vi "Save_Data.vi"(1 "Index":u16, 2 "Plot Type":T1=enum."Voltage trace") -> ()   [LabVIEW 2016]
uses:
  Controls/Graph_Type.ctl
  Controls/XY_Plot_Cluster.ctl
  Controls/Inst_type.ctl
  Globals/Meas_global.vi
  Globals/Plug_in_data_global.vi
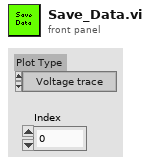
[diagram p1: front panel]
types:
  T1 = typedef "Graph_Type.ctl" = enum16{"Show no graph", "Voltage trace", "Velocity trace", "Vel histogram", "Spectrum", "f.E(f) v Log f", "Auto-Corr"}
  T2 = typedef "Analysis_info_cluster.ctl" = cluster{"Colour":u32, "Inst type":T3, "Inst name":string, "Symbol":string, "Code name":string, "Extra Info":string, "Inst Array":T4, "Extra Titles":string[], "Extra Values":string[], "U":dbl, "u^2":dbl, "u^3":dbl, "u^4":dbl, "Skew_u":dbl, "Kurt_u":dbl, "Sd Error in Mean":dbl, "% u'/U":dbl, "X":dbl, "Y":dbl, "Z":dbl, "Timescale integral Estimate":dbl, "Sd Error in Variance":dbl, "Calib File":path, "Calib Constants":dbl[], "Output Position":bool, "Full Stats":bool, "Av Sampling Rate":dbl, "Av No of Samples":dbl, "Total Meas Time (s)":dbl, "ADAM Ch Name":string, "Max value":dbl, "Min value":dbl}
  T3 = typedef "Inst_type.ctl" = enum16{"Propeller anemometer", "Raw voltage", "Pressure Transducer", "Pitot-static tube", "Preston tube", "Hot wire", "Cross wire 1", "Cross wire 2", "Generic Linear", "Generic Polynomial", "Generic BackPoly", "Fast FID", "Thermocouple", "Cold wire", "Pulsed Wire", "LDA Vel", "LDA Tran time", "LDA Arr time", "Microphone"}
  T4 = typedef "Instrument_Array.ctl" = enum16{"PWA", "LDA", "Analogue"}
  T5 = typedef "Post_Process.ctl" = enum16{"Take New Data", "Post Process Raw Data File"}
  T6 = typedef "XY_Plot_Cluster.ctl" = cluster{"First Name":string, "Second Name":string, "X axis name":string, "Y axis name":string, "X array":dbl[], "Y array":dbl[], "Weighting":dbl[]}
  T7 = typedef "Time_Trace_Cluster.ctl" = cluster{"Weighting":dbl[], "Time (s)":dbl[], "Voltage":dbl[], "Eng Values":dbl[]}
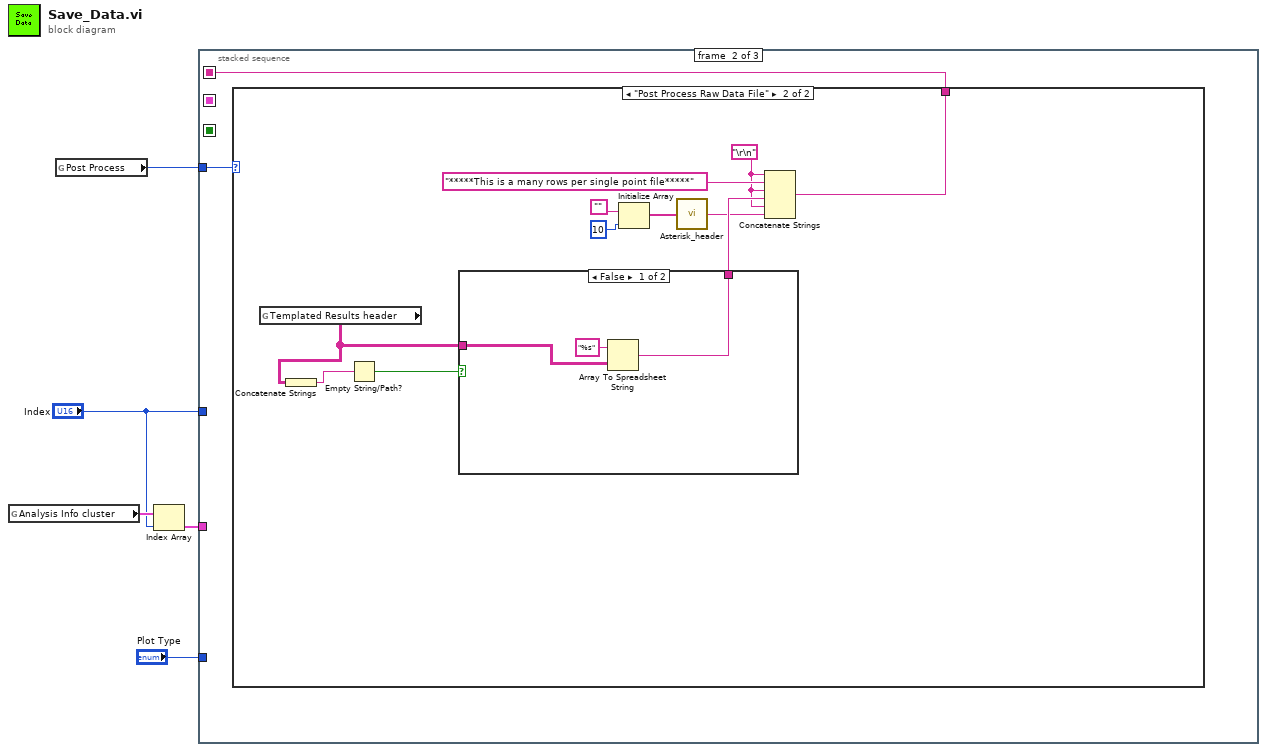
[diagram p0: block diagram]
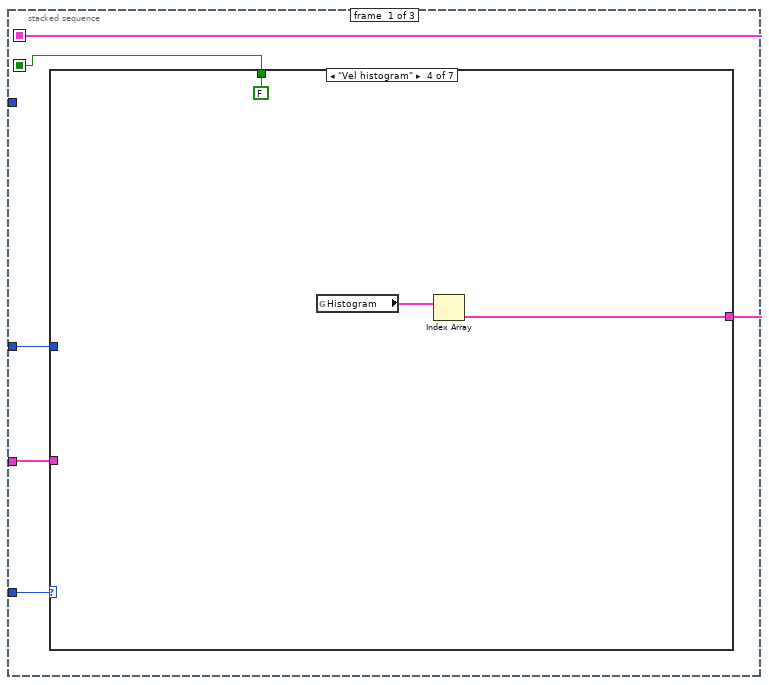
[diagram p2: hidden frame]
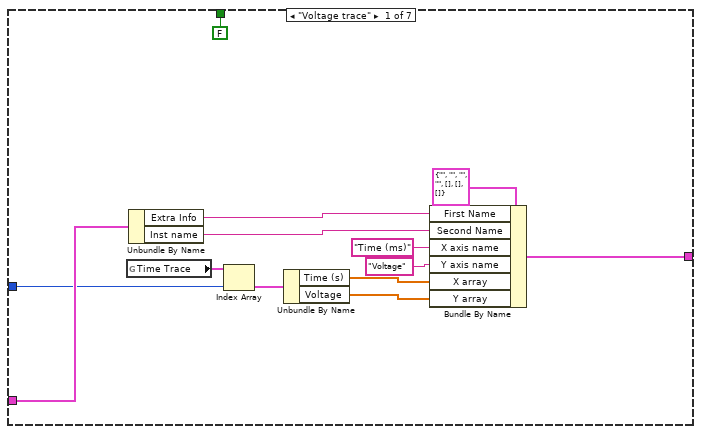
[diagram p3: hidden frame]
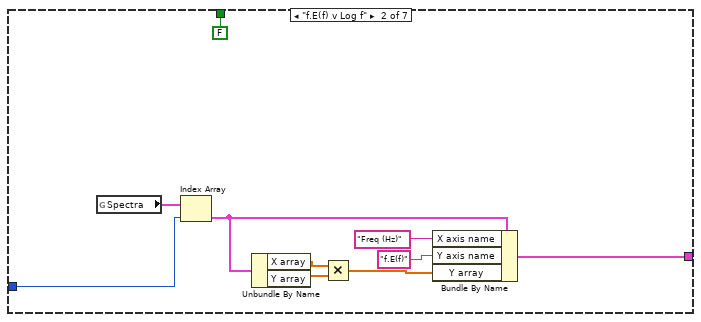
[diagram p4: hidden frame]
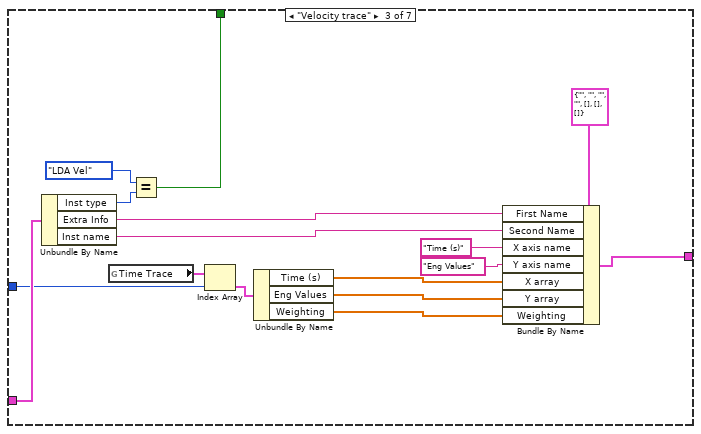
[diagram p5: hidden frame]
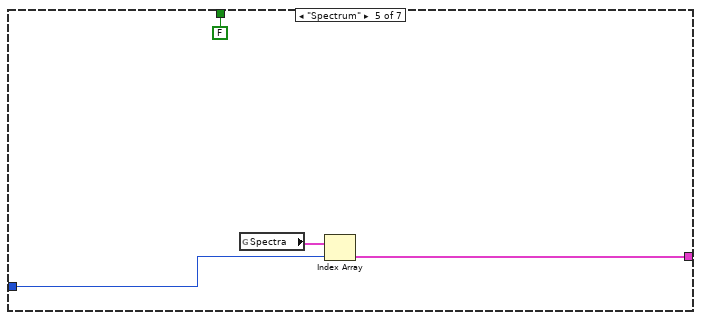
[diagram p6: hidden frame]
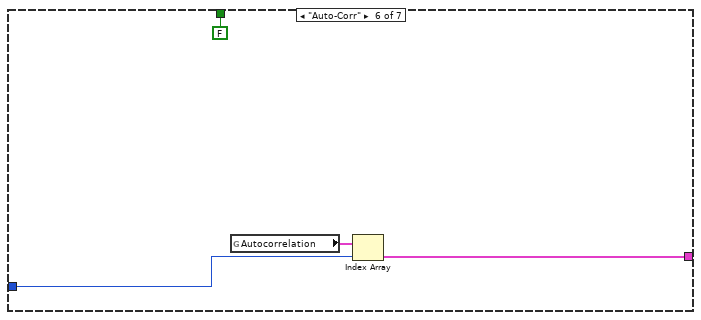
[diagram p7: hidden frame]
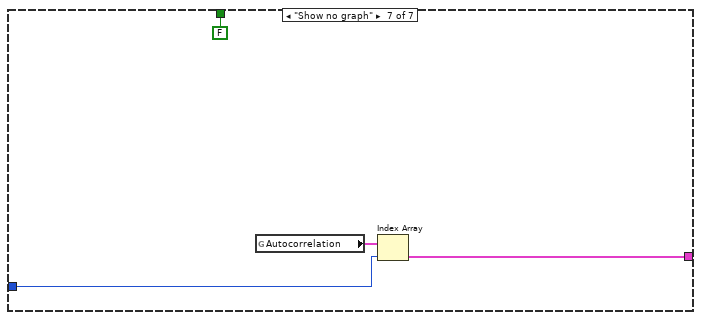
[diagram p8: hidden frame]
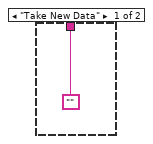
[diagram p9: hidden frame]
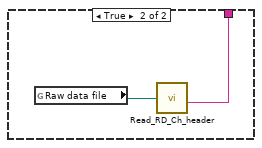
[diagram p10: hidden frame]
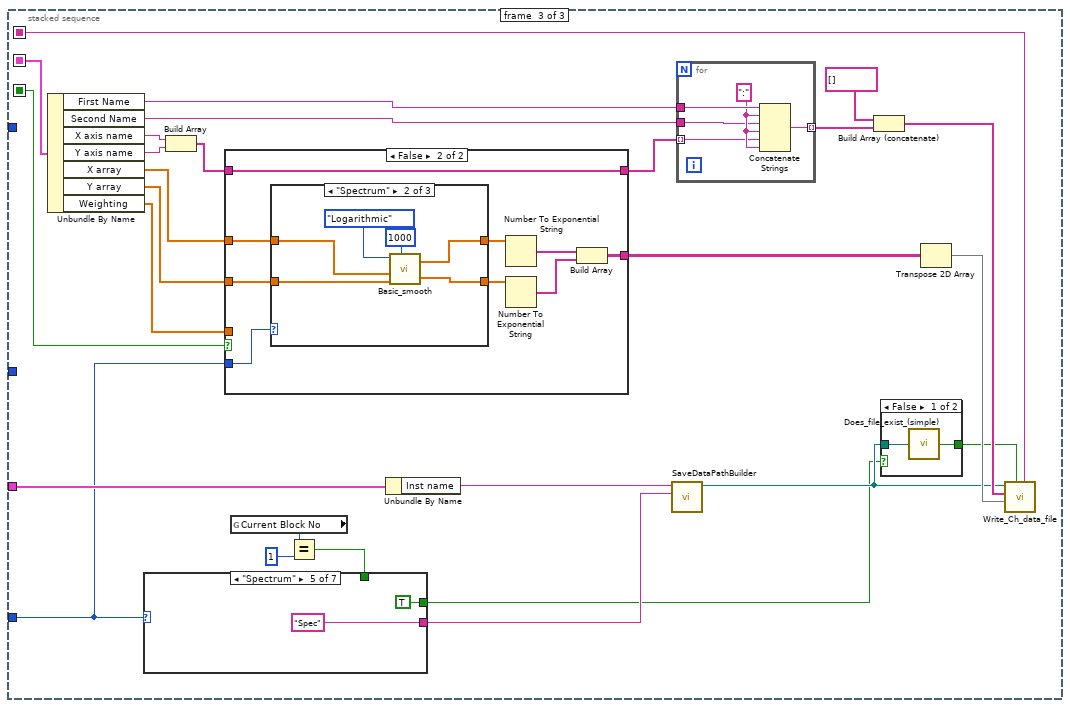
[diagram p11: hidden frame]
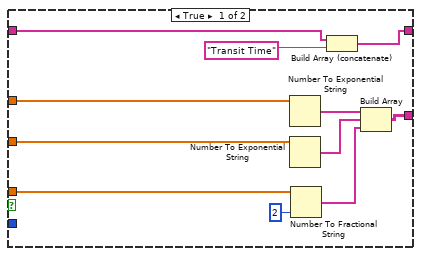
[diagram p12: hidden frame]
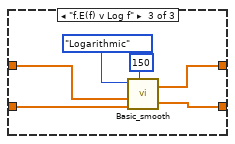
[diagram p14: hidden frame]
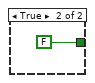
[diagram p15: hidden frame]
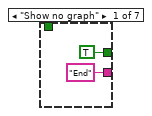
[diagram p16: hidden frame]
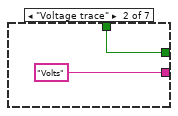
[diagram p17: hidden frame]
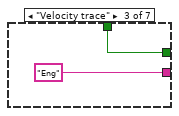
[diagram p18: hidden frame]
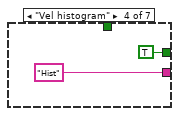
[diagram p19: hidden frame]
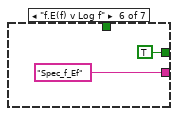
[diagram p20: hidden frame]
diagram:
  n1 = global read "Meas_global.vi" "Analysis Info cluster"() -> (w3:T2[])
  n2 = global read "Meas_global.vi" "Post Process"() -> (w4:T5)
  n3 = Index Array(array=w3, index="Index") -> (element=w2:T2)
  n4 = stacked-sequence {
    seq-local: [w8 _ _] -> [_ _ w95]
    seq-local: [_ w65 _] -> [_ _ w96]
    seq-local: [w6 _ _] -> [_ _ w91]
    tunnel: "Plot Type" -> [w10 _ w94]
    tunnel: w2 -> [w9 _ w104]
    tunnel: w4 -> [_ w66 _]
    tunnel: "Index" -> [w7 _ _]
    frame #0 {
      n5 = case shown="\"Vel histogram\"" w10 {
        tunnel: w9 -> [w23 _ w49 _ _ _ _]
        tunnel: [w18 w31 w44 w51 w56 w58 w62] -> w8
        tunnel: w7 -> [w16 w26 w41 _ w55 w59 w63]
        tunnel: [FALSE FALSE w34 FALSE FALSE FALSE FALSE] -> w6
        frame "Voltage trace" {
          n6 = global read "Meas_global.vi" "Time Trace"() -> (w17:T7[])
          n7 = Unbundle By Name(w23) -> ("Extra Info"=w22:string, "Inst name"=w21:string)
          n8 = Index Array(array=w17, index=w16) -> (element=w15:T7)
          n9 = Unbundle By Name(w15) -> ("Time (s)"=w14:dbl[], "Voltage"=w13:dbl[])
          n10 = Bundle By Name(cluster=T6 {"First Name"="", "Second Name"="", "X axis name"="", "Y axis name"="", "X array"=[], "Y array"=[], "Weighting"=[]} ("Spectra"), "First Name"=w22, "Second Name"=w21, "X axis name"="Time (ms)", "Y axis name"="Voltage", "X array"=w14, "Y array"=w13) -> (w18:T6)
        }
        frame "f.E(f) v Log f" {
          n11 = global read "Meas_global.vi" "Spectra"() -> (w27:T6[])
          n12 = Index Array(array=w27, index=w26) -> (element=w25:T6)
          n13 = Unbundle By Name(w25) -> ("X array"=w29:dbl[], "Y array"=w30:dbl[])
          n14 = Multiply(x=w29, y=w30) -> (x*y=w28:dbl[])
          n15 = Bundle By Name(cluster=w25, "X axis name"="Freq (Hz)", "Y axis name"="f.E(f)", "Y array"=w28) -> (w31:T6)
        }
        frame "Velocity trace" {
          n16 = Unbundle By Name(w49) -> ("Inst type"=w36:T3, "Extra Info"=w48:string, "Inst name"=w47:string)
          n17 = global read "Meas_global.vi" "Time Trace"() -> (w42:T7[])
          n18 = Equal?(x=Inst_type."LDA Vel" ("Inst type"), y=w36) -> (x = y?=w34:bool)
          n19 = Index Array(array=w42, index=w41) -> (element=w40:T7)
          n20 = Unbundle By Name(w40) -> ("Time (s)"=w39:dbl[], "Eng Values"=w38:dbl[], "Weighting"=w37:dbl[])
          n21 = Bundle By Name(cluster=T6 {"First Name"="", "Second Name"="", "X axis name"="", "Y axis name"="", "X array"=[], "Y array"=[], "Weighting"=[]} ("Spectra"), "First Name"=w48, "Second Name"=w47, "X axis name"="Time (s)", "Y axis name"="Eng Values", "X array"=w39, "Y array"=w38, "Weighting"=w37) -> (w44:T6)
        }
        frame "Vel histogram" {
          n22 = global read "Meas_global.vi" "Histogram"() -> (w52:T6[])
          n23 = Index Array(array=w52) -> (element=w51:T6)  [unwired: 1 in]
        }
        frame "Spectrum" {
          n24 = global read "Meas_global.vi" "Spectra"() -> (w54:T6[])
          n25 = Index Array(array=w54, index=w55) -> (element=w56:T6)
        }
        frame "Auto-Corr" {
          n26 = global read "Meas_global.vi" "Autocorrelation"() -> (w60:T6[])
          n27 = Index Array(array=w60, index=w59) -> (element=w58:T6)
        }
        frame "Show no graph" {
          n28 = global read "Meas_global.vi" "Autocorrelation"() -> (w64:T6[])
          n29 = Index Array(array=w64, index=w63) -> (element=w62:T6)
        }
      }
    }
    frame #1 {
      n30 = case shown="\"Post Process Raw Data File\"" w66 {
        tunnel: ["" w70] -> w65
        frame "Take New Data" {
        }
        frame "Post Process Raw Data File" {
          w71 = "\r\n"
          n31 = global read "Plug_in_data_global.vi" "Templated Results header"() -> (w69:string[][])
          n32 = Concatenate Strings(w69) -> (w68:string)
          n33 = Empty String/Path?(string/path=w68) -> (empty?=w77:bool)
          n34 = case shown="False" w77 {
            tunnel: [w79 w82] -> w76
            tunnel: w69 -> [w80 _]
            frame False {
              n35 = Array To Spreadsheet String(array=w80, 3:"%s" ("format string")) -> (spreadsheet string=w79:string)  [unwired: 1 out]
            }
            frame True {
              n36 = global read "Meas_global.vi" "Raw data file"() -> (w83:path)
              n37 = call "Read_RD_Ch_header.vi"("Raw data file"=w83) -> ("Ch string"=w82:string)  [unwired: 3 out]
            }
          }
          n38 = Initialize Array("", 10) -> (w75:string[])
          n39 = call "Asterisk_header.vi"("Channel names"=w75) -> ("Header string"=w72:string)
          n40 = Concatenate Strings(w71, "*****This is a many rows per single point file*****", w71, w76, w71, w72) -> (w70:string)
        }
      }
    }
    frame #2 {
      n41 = Unbundle By Name(w95) -> ("First Name"=w106:string, "Second Name"=w89:string, "X axis name"=w87:string, "Y axis name"=w86:string, "X array"=w93:dbl[], "Y array"=w92:dbl[], "Weighting"=w90:dbl[])
      n42 = Build Array(w87, w86) -> (w84:string[])
      n43 = case shown="False" w91 {
        tunnel: [w126 w135] -> w107
        tunnel: w94 -> [_ w133]
        tunnel: w93 -> [w124 w132]
        tunnel: w92 -> [w123 w131]
        tunnel: w90 -> [w121 _]
        tunnel: [w118 w127] -> w85
        tunnel: w84 -> [w119 w127]
        frame True {
          n44 = Number To Exponential String(number=w124) -> (E-format string=w122:string[])  [unwired: 3 in]
          n45 = Number To Exponential String(number=w123) -> (E-format string=w125:string[])  [unwired: 3 in]
          n46 = Number To Fractional String(number=w121, precision (6)=i16 2) -> (F-format string=w120:string[])  [unwired: 2 in]
          n47 = Build Array (concatenate)(w119, "Transit Time") -> (w118:string[])
          n48 = Build Array(w122, w125, w120) -> (w126:string[][])
        }
        frame False {
          n49 = case shown="\"Spectrum\"" w133 {
            tunnel: [w137 w141 w147] -> w129
            tunnel: w132 -> [w137 w143 w149]
            tunnel: w131 -> [w136 w142 w148]
            tunnel: [w136 w140 w146] -> w130
            frame "Voltage trace", Default {
            }
            frame "Spectrum" {
              n50 = call "Basic_smooth.vi"("Smoothing"=enum16{"Linear", "Logarithmic"}."Logarithmic", "X array in"=w143, "Y array in"=w142, "No of estimates output"=1000) -> ("X array Out"=w141:dbl[], "Y array Out"=w140:dbl[])  [unwired: 1 out]
            }
            frame "f.E(f) v Log f" {
              n51 = call "Basic_smooth.vi"("Smoothing"=enum16{"Linear", "Logarithmic"}."Logarithmic", "X array in"=w149, "Y array in"=w148, "No of estimates output"=150) -> ("X array Out"=w147:dbl[], "Y array Out"=w146:dbl[])  [unwired: 1 out]
            }
          }
          n52 = Number To Exponential String(number=w129) -> (E-format string=w128:string[])  [unwired: 3 in]
          n53 = Number To Exponential String(number=w130) -> (E-format string=w134:string[])  [unwired: 3 in]
          n54 = Build Array(w128, w134) -> (w135:string[][])
        }
      }
      n55 = global read "Meas_global.vi" "Current Block No"() -> (w100:i32)
      n56 = Equal?(x=w100, y=1) -> (x = y?=w97:bool)
      n57 = case shown="\"Spectrum\"" w94 {
        tunnel: ["End" "Volts" "Eng" "Hist" "Spec" "Spec_f_Ef" "Auto"] -> w105
        tunnel: [TRUE w155 w157 TRUE TRUE TRUE TRUE] -> w98
        tunnel: w97 -> [_ w155 w157 _ _ _ _]
        frame "Show no graph" {
        }
        frame "Voltage trace" {
        }
        frame "Velocity trace" {
        }
        frame "Vel histogram" {
        }
        frame "Spectrum" {
        }
        frame "f.E(f) v Log f" {
        }
        frame "Auto-Corr" {
        }
      }
      n58 = Unbundle By Name(w104) -> ("Inst name"=w103:string)
      n59 = call "SaveDataPathBuilder.vi"("DataTypeSuffix"=w105, "Inst name"=w103) -> ("Path name Out"=w101:path)  [unwired: 9 in]
      n60 = for {
        tunnel: w106 -> [w115]
        tunnel: w89 -> [w113]
        tunnel: [w112] -> w88 mode=indexing
        tunnel: w85 -> [w111] mode=indexing
        w114 = ":" ("string")
        n61 = Concatenate Strings(w115, w114, w113, w114, w111, w114) -> (w112:string)
      }
      n62 = Build Array (concatenate)(string[] [], w88) -> (w109:string[])
      n63 = case shown="False" w98 {
        tunnel: [w151 FALSE] -> w102
        tunnel: w101 -> [w150 _]
        frame False {
          n64 = call "Does_file_exist_(simple).vi"("Pathname"=w150) -> ("exists?"=w151:bool)
        }
        frame True {
        }
      }
      n65 = Transpose 2D Array(2D array=w107) -> (transposed array=w108:string[][])
      n66 = call "Write_Ch_data_file.vi"("Header string"=w96, "exists?"=w102, "Channel Values"=w108, "Channel names"=w109, "Filename"=w101) -> ()  [unwired: 2 in, 5 out]
    }
  }
